vi "Configure Autozero.vi"(8 "error in (no error)":errorcluster, 10 "Autozero  (0: On)":u16(ring) items=["On", "Off", "Once"], 11 "VISA resource name":refnum<visa-resource-name>) -> (0 "error out":errorcluster, 3 "VISA resource name out":refnum<visa-resource-name>)   [LabVIEW 2010, in "Keithley 24XX.lvlib"]
doc: "Enables or disables the autozero function on the instrument. Enabling autozero optimizes the instrument for accuracy, while disabling optimizes for speed."
uses:
  <instrlib>/Keithley 24XX/Keithley 24XX.lvlib
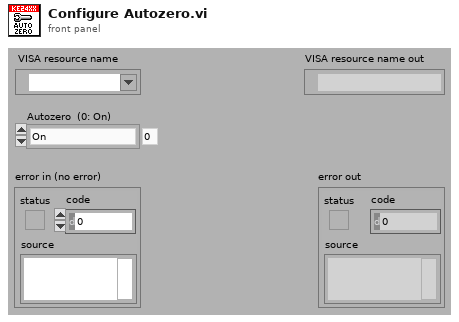
[diagram p1: front panel]
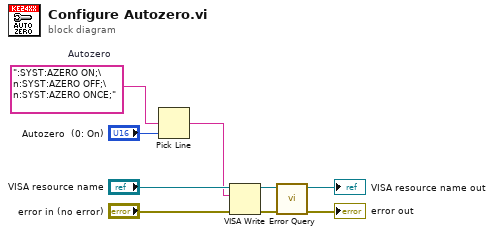
[diagram p0: block diagram]
diagram:
  w1 = ":SYST:AZERO ON;\n:SYST:AZERO OFF;\n:SYST:AZERO ONCE;"  # Autozero
  n1 = Pick Line(multi-line string=w1, line index="Autozero  (0: On)") -> (output string=w3:string)  [unwired: 1 in]
  n2 = VISA Write(VISA resource name="VISA resource name", write buffer=w3, error in (no error)="error in (no error)") -> (VISA resource name out=w5:refnum<visa-resource-name>, error out=w4:errorcluster)  [unwired: 1 out]
  n3 = call <instrlib>:"Error Query.vi"("error in (no error)"=w4, "VISA resource name"=w5) -> ("error out"=→"error out":errorcluster, "VISA resource name out"=→"VISA resource name out":refnum<visa-resource-name>)  [unwired: 6 in, 2 out]
